vi "Calculation steps for partial mode (SILAR).vi"(0 "Loop iteration для кол-ва циклов":i32, 1 "Кол-во жидкости в каждом стакане [мм]":dbl, 2 "Высота стакана [мм]":dbl=81.2, 3 "Высота подложки [мм]":dbl, 4 "Loop iteration для кол-ва используемых растворов":i32, 5 "Loop iteration для кол-ва погружений в каждый стакан":i32) -> (14 "Кол-во шагов до раствора":dbl, 19 "Кол-во шагов над раствором":dbl)   [LabVIEW 2016]
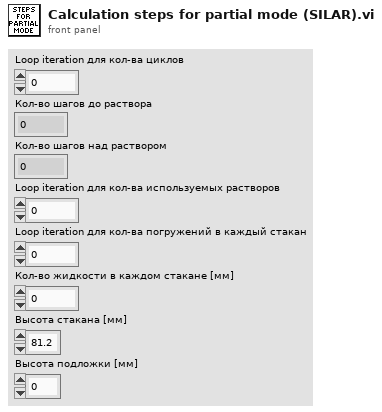
[diagram p1: front panel]
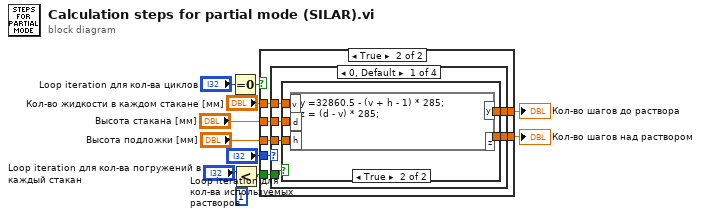
[diagram p0: block diagram]
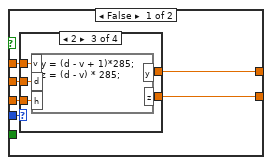
[diagram p2: hidden frame]
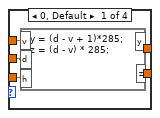
[diagram p3: hidden frame]
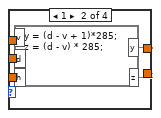
[diagram p4: hidden frame]
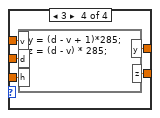
[diagram p5: hidden frame]
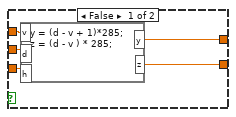
[diagram p6: hidden frame]
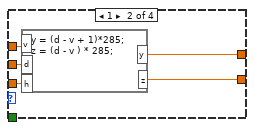
[diagram p7: hidden frame]
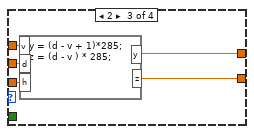
[diagram p8: hidden frame]
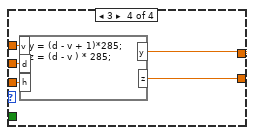
[diagram p9: hidden frame]
diagram:
  n1 = Equal To 0?(x="Loop iteration для кол-ва циклов") -> (x = 0?=w3:bool)
  n2 = Less?(x="Loop iteration для кол-ва погружений в каждый стакан", y=1) -> (x < y?=w10:bool)
  n3 = case shown="True" w3 {
    tunnel: "Кол-во жидкости в каждом стакане [мм]" -> [w17 w44]
    tunnel: "Высота подложки [мм]" -> [w15 w43]
    tunnel: [w13 w42] -> w5
    tunnel: "Loop iteration для кол-ва используемых растворов" -> [w14 w40]
    tunnel: "Высота стакана [мм]" -> [w16 w39]
    tunnel: [w12 w41] -> w4
    tunnel: w10 -> [_ w38]
    frame False {
      n4 = case shown="2" w14 {
        tunnel: w17 -> [w22 w27 w32 w37]
        tunnel: w15 -> [w21 w26 w30 w35]
        tunnel: [w20 w25 w29 w34] -> w13
        tunnel: [w19 w24 w28 w33] -> w12
        tunnel: w16 -> [w18 w23 w31 w36]
        frame 0, Default {
          n5 = formula code="y = (d - v + 1)*285;\nz = (d - v) * 285;"("v"=w22, "h"=w21, "d"=w18) -> ("y"=w20:dbl, "z"=w19:dbl)
        }
        frame 1 {
          n6 = formula code="y = (d - v + 1)*285;\nz = (d - v) * 285;"("v"=w27, "h"=w26, "d"=w23) -> ("y"=w25:dbl, "z"=w24:dbl)
        }
        frame 2 {
          n7 = formula code="y = (d - v + 1)*285;\nz = (d - v) * 285;"("v"=w32, "h"=w30, "d"=w31) -> ("y"=w29:dbl, "z"=w28:dbl)
        }
        frame 3 {
          n8 = formula code="y = (d - v + 1)*285;\nz = (d - v) * 285;"("v"=w37, "h"=w35, "d"=w36) -> ("y"=w34:dbl, "z"=w33:dbl)
        }
      }
    }
    frame True {
      n9 = case shown="0, Default" w40 {
        tunnel: w44 -> [w50 w65 w70 w75]
        tunnel: w43 -> [w49 w64 w68 w73]
        tunnel: [w48 w63 w67 w72] -> w42
        tunnel: [w47 w62 w66 w71] -> w41
        tunnel: w39 -> [w45 w61 w69 w74]
        tunnel: w38 -> [w46 _ _ _]
        frame 0, Default {
          n10 = case shown="True" w46 {
            tunnel: w50 -> [w55 w60]
            tunnel: w49 -> [w53 w59]
            tunnel: [w52 w58] -> w48
            tunnel: [w51 w57] -> w47
            tunnel: w45 -> [w54 w56]
            frame False {
              n11 = formula code="y = (d - v + 1)*285;\nz = (d - v ) * 285;"("v"=w55, "h"=w53, "d"=w54) -> ("y"=w52:dbl, "z"=w51:dbl)
            }
            frame True {
              n12 = formula code="y =32860.5 - (v + h - 1) * 285;\nz = (d - v) * 285;"("v"=w60, "h"=w59, "d"=w56) -> ("y"=w58:dbl, "z"=w57:dbl)
            }
          }
        }
        frame 1 {
          n13 = formula code="y = (d - v + 1)*285;\nz = (d - v ) * 285;"("v"=w65, "h"=w64, "d"=w61) -> ("y"=w63:dbl, "z"=w62:dbl)
        }
        frame 2 {
          n14 = formula code="y = (d - v + 1)*285;\nz = (d - v ) * 285;"("v"=w70, "h"=w68, "d"=w69) -> ("y"=w67:dbl, "z"=w66:dbl)
        }
        frame 3 {
          n15 = formula code="y = (d - v + 1)*285;\nz = (d - v ) * 285;"("v"=w75, "h"=w73, "d"=w74) -> ("y"=w72:dbl, "z"=w71:dbl)
        }
      }
    }
  }
  "Кол-во шагов до раствора" <- w5
  "Кол-во шагов над раствором" <- w4
